vi "_Do Pause Feature.vi"   [LabVIEW 2012]
uses:
  <vilib>/rvi/DataTransferAndStorage/Container/Common/niFpgaContainerGetUniqueNameForEmu.vi
  <vilib>/rvi/Memory/Memory_Emulation/niFpgaMemoryEmulationCacheClearOnFirstRun.vi
  <vilib>/rvi/Memory/Memory_Emulation/nirvimemoryEmulationManagerCache_MakeExclusive.vi
  <vilib>/rvi/Memory/Memory_Emulation/niFpgaMemoryEmulationValidateCache.vi
  <vilib>/rvi/Memory/Memory_Emulation/nirvimemoryEmulationManagerCache_ReleaseExclusive.vi
  <vilib>/rvi/Memory/Memory_Emulation/nirvimemoryEmulationManagerCache_InsertValue.vi
  <vilib>/Utility/error.llb/Clear Errors.vi
  <vilib>/rvi/Memory/Memory_Emulation/nirvimemoryEmulationManagerCache_GetValue.vi
  <vilib>/rvi/DataTransferAndStorage/Container/XNode/niFpgaContainer.xnode
  <vilib>/rvi/Memory/Memory_Emulation/nirvimemoryEmulation.vi
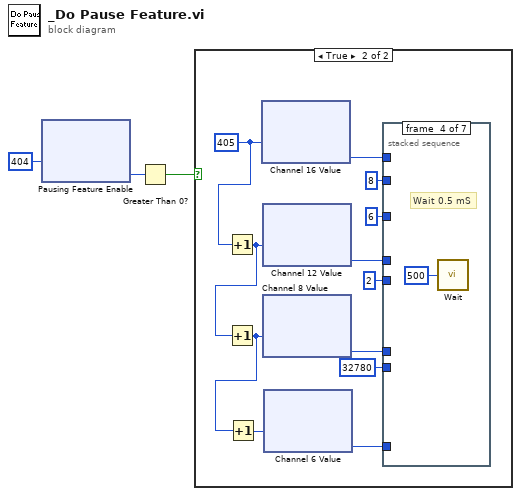
[diagram p0: block diagram]
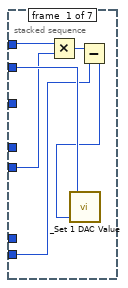
[diagram p3: hidden frame]
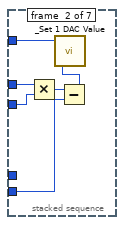
[diagram p4: hidden frame]
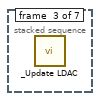
[diagram p5: hidden frame]
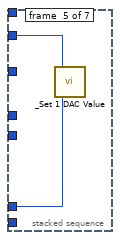
[diagram p6: hidden frame]
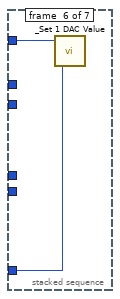
[diagram p7: hidden frame]
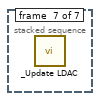
[diagram p8: hidden frame]
diagram:
  n1 = xnode "Pausing Feature Enable"("Address"=u32 404) -> ("Data"=w3:u32)  [unwired: 1 in, 1 out]
  n2 = Greater Than 0?(x=w3) -> (x > 0?=w1:bool)
  n3 = case shown="True" w1 {
    frame False {
    }
    frame True {
      w15 = u32 405 ("Address")
      n4 = Increment(x=w15) -> (x+1=w13:u32)
      n5 = Increment(x=w13) -> (x+1=w12:u32)
      n6 = Increment(x=w12) -> (x+1=w14:u32)
      n7 = xnode "Channel 16 Value"("Address"=w15) -> ("Data"=w11:u32)  [unwired: 1 in, 1 out]
      n8 = xnode "Channel 12 Value"("Address"=w13) -> ("Data"=w10:u32)  [unwired: 1 in, 1 out]
      n9 = xnode "Channel 8 Value"("Address"=w12) -> ("Data"=w9:u32)  [unwired: 1 in, 1 out]
      n10 = xnode "Channel 6 Value"("Address"=w14) -> ("Data"=w8:u32)  [unwired: 1 in, 1 out]
      n11 = stacked-sequence {
        tunnel: w11 -> [w20 _ _ _ _ _ _]
        tunnel: w10 -> [_ w23 _ _ _ _ _]
        tunnel: w9 -> [_ _ _ _ w29 _ _]
        tunnel: w8 -> [_ _ _ _ _ w31 _]
        tunnel: u8 8 ("Ch#") -> [w21 _ _ _ w30 _ _]
        tunnel: u8 6 ("Ch#") -> [_ w27 _ _ _ w32 _]
        tunnel: u32 2 ("Ch#") -> [w19 w25 _ _ _ _ _]
        tunnel: u32 32780 ("Ch#") -> [w17 w24 _ _ _ _ _]
        frame #0 {
          n12 = Multiply(x=w20, y=w19) -> (x*y=w18:u32)
          n13 = Subtract(x=w18, y=w17) -> (x-y=w16:u32)
          n14 = call "_Set 1 DAC Value.vi"("DAC"=w16, "Ch#"=w21) -> ()  [unwired: 2 out]
        }
        frame #1 {
          n15 = Multiply(x=w23, y=w25) -> (x*y=w26:u32)
          n16 = Subtract(x=w26, y=w24) -> (x-y=w22:u32)
          n17 = call "_Set 1 DAC Value.vi"("DAC"=w22, "Ch#"=w27) -> ()  [unwired: 2 out]
        }
        frame #2 {
          n18 = call "_Update LDAC.vi"() -> ()  [unwired: 6 out]
        }
        frame #3 {
          # "Wait 0.5 mS"
          n19 = call "Wait"("Count(uSec)"=u16 500) -> ()  [unwired: 1 out]
        }
        frame #4 {
          n20 = call "_Set 1 DAC Value.vi"("DAC"=w29, "Ch#"=w30) -> ()  [unwired: 2 out]
        }
        frame #5 {
          n21 = call "_Set 1 DAC Value.vi"("DAC"=w31, "Ch#"=w32) -> ()  [unwired: 2 out]
        }
        frame #6 {
          n22 = call "_Update LDAC.vi"() -> ()  [unwired: 6 out]
        }
      }
    }
  }
